vi "Format PlacementResponseType_LVXML.vi"(8 "error in (no error)":errorcluster, 10 "valueXmlData in":T2, 11 "AWS_EC2 in":refnum<class "AWS_EC2.lvclass">) -> (0 "error out":errorcluster, 2 "PlacementResponseType":T3, 3 "AWS_EC2 out":refnum<class "AWS_EC2.lvclass">)   [LabVIEW 2014, in "AWS_EC2.lvlib" / "AWS_EC2.lvclass"]
uses:
  AWS_EC2.lvclass
  EC2 Datatypes/PlacementResponseType.ctl
  lv-xml-parser/r0/trunk/VI Source/EventType.ctl
  AWS_EC2.lvlib
  lv-xml-parser/r0/trunk/VI Source/LV XML Parser.lvlib
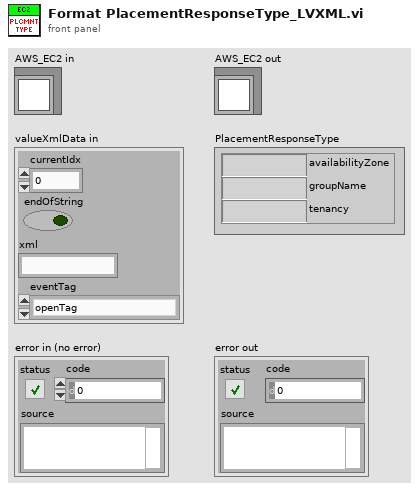
[diagram p1: front panel]
types:
  T1 = typedef "LV XML Parser.lvlib/EventType.ctl" = enum16{"openTag", "endOpenTag", "closeTag", "comment", "endComment", "endOfFile", "attribute", "startXml"}
  T2 = cluster{"currentIdx":i32, "endOfString":bool, "xml":string, "eventTag":T1}
  T3 = typedef "AWS_EC2.lvlib/PlacementResponseType.ctl" = cluster{"availabilityZone":string, "groupName":string, "tenancy":string}
  T4 = cluster{"namespaceUri":string, "localName":string}
  T5 = cluster{"Attributes":cluster{"localName":string, "namespaceUri":string, "value":string}[], "localName":string, "namespaceUri":string, "valueXmlData":cluster{"currentIdx":i32, "endOfString":bool, "xml":string, "eventTag":T1}}[]
  T6 = cluster{"Attributes":cluster{"localName":string, "namespaceUri":string, "value":string}[], "localName":string, "namespaceUri":string, "valueXmlData":cluster{"currentIdx":i32, "endOfString":bool, "xml":string, "eventTag":T1}}
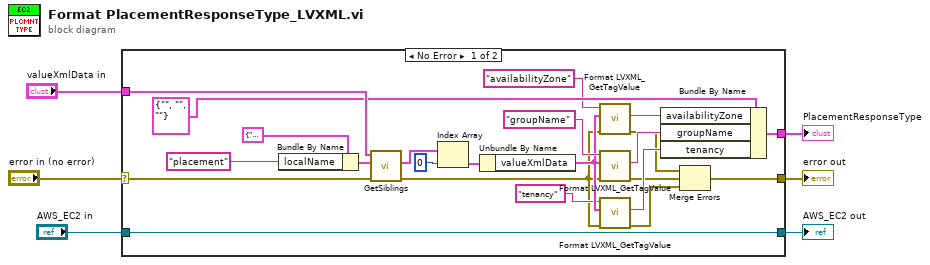
[diagram p0: block diagram]
diagram:
  n1 = case shown="No Error" "error in (no error)" {
    selector: "error in (no error)" -> [w25 w30]
    tunnel: [w24 w31] -> w4
    tunnel: "AWS_EC2 in" -> [w24 w31]
    tunnel: [w10 w30] -> w2
    tunnel: "valueXmlData in" -> [w29 _]
    tunnel: [w22 _] -> w6
    frame No Error {
      n2 = Bundle By Name(cluster=T4 {"namespaceUri"="", "localName"=""} ("limitToTag"), "localName"="placement" ("Tag name")) -> (w26:T4)
      n3 = call "GetSiblings.vi"("error in (no error)"=w25, "limitToTag"=w26, "xmlData"=w29) -> ("error out"=w13:errorcluster, "Siblings"=w17:T5)  [unwired: 7 in]
      n4 = Index Array(array=w17, index=0) -> (element=w18:T6)
      n5 = Unbundle By Name(w18) -> ("valueXmlData"=w15:T2)
      n6 = call "Format LVXML_GetTagValue.vi"("error in (no error)"=w13, "xmlDataIn"=w15, "Tag name"="availabilityZone") -> ("error out"=w9:errorcluster, "Value"=w20:string)  [unwired: 6 in, 1 out]
      n7 = call "Format LVXML_GetTagValue.vi"("error in (no error)"=w13, "xmlDataIn"=w15, "Tag name"="groupName") -> ("error out"=w8:errorcluster, "Value"=w11:string)  [unwired: 6 in, 1 out]
      n8 = call "Format LVXML_GetTagValue.vi"("error in (no error)"=w13, "xmlDataIn"=w15, "Tag name"="tenancy") -> ("error out"=w7:errorcluster, "Value"=w12:string)  [unwired: 6 in, 1 out]
      n9 = Bundle By Name(cluster=T3 {"availabilityZone"="", "groupName"="", "tenancy"=""} ("PlacementResponseType"), "availabilityZone"=w20, "groupName"=w11, "tenancy"=w12) -> (w22:T3)
      n10 = Merge Errors(w9, w8, w7) -> (w10:errorcluster)
    }
    frame Error {
    }
  }
  "PlacementResponseType" <- w6
  "AWS_EC2 out" <- w4
  "error out" <- w2
